vi "Launch Debugging.vi"(8 "error in (no error)":errorcluster, 10 "Parent In":refnum<class "Module.lvclass">, 11 "Debug Launcher in":refnum<class "Debug Launcher.lvclass">) -> (0 "error out":errorcluster, 2 "Parent":refnum<class "Module.lvclass">)   [LabVIEW 2020, in "Volatus.lvlib" / "Debug Launcher.lvclass"]
uses:
  Debug Launcher.lvclass
  Module/Module.lvclass
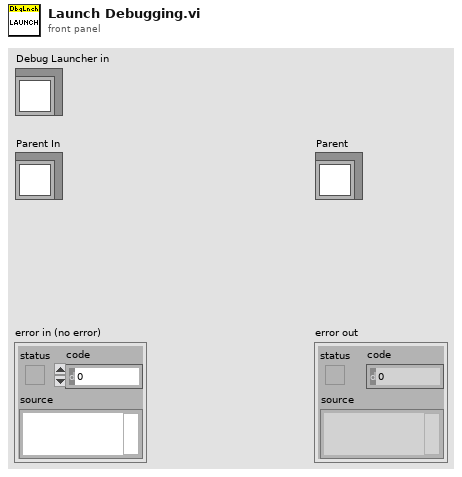
[diagram p1: front panel]
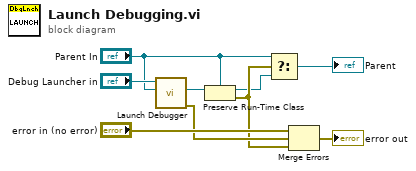
[diagram p0: block diagram]
diagram:
  n1 = call-dynamic "Launch Debugger.vi"("Parent In"="Parent In", "Debug Launcher in"="Debug Launcher in") -> ("error out"=w5:errorcluster, "Parent"=w7:refnum<class "Module.lvclass">)  [unwired: 8 in]
  n2 = Preserve Run-Time Class(object in=w7, 2:"Parent In") -> (object out=w2:refnum<class "Module.lvclass">, error out=w3:errorcluster)  [unwired: 1 in]
  n3 = Select(t="Parent In", s=w3, f=w2) -> (s? t:f=→"Parent":refnum<class "Module.lvclass">)
  n4 = Merge Errors("error in (no error)", w5, w3) -> (→"error out":errorcluster)
